vi "Can软件版本号.vi"() -> (3 "软件版本号":string)   [LabVIEW 2020]
uses:
  Libraries/ZLG_CAN/ZLG_CAN.lvlib
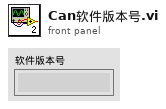
[diagram p1: front panel]
types:
  T1 = typedef "ZLG_CAN.lvlib/CAN_Frame.ctl" = cluster{"[0]":u8, "[1]":u8, "[2]":u8, "[3]":u8, "[4]":u8, "[5]":u8, "[6]":u8, "[7]":u8}
  T2 = typedef "ZLG_CAN.lvlib/Sent_Recive (Reply Payload)--cluster.ctl" = cluster{"Receive":T3[], "Sent_Recive_error":errorcluster}
  T3 = typedef "ZLG_CAN.lvlib/CAN_OBJ_R.ctl" = cluster{"ID":u32, "TimeStamp":u32, "TimeFlag":u8, "SendType":u8, "RemoteFlag":u8, "ExternFlag":u8, "DataLen":u8, "数值":u8, "数值":u8, "数值":u8, "数值":u8, "数值":u8, "数值":u8, "数值":u8, "数值":u8, "数值":u8, "数值":u8, "数值":u8}
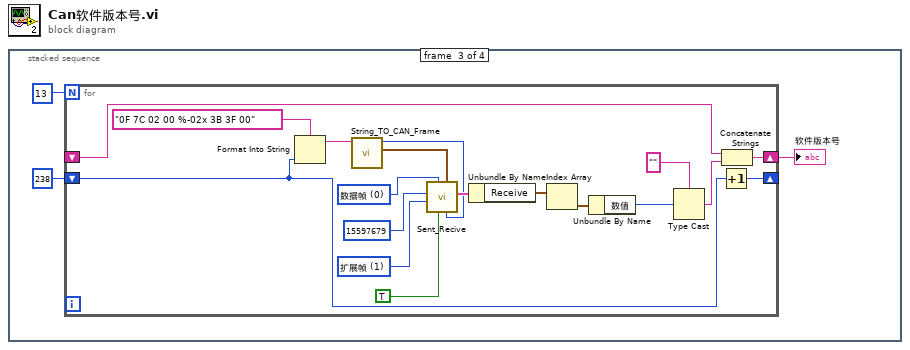
[diagram p0: block diagram]
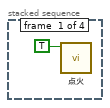
[diagram p2: hidden frame]
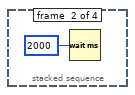
[diagram p3: hidden frame]
diagram:
  n1 = stacked-sequence {
    frame #0 {
      n2 = call "点火.vi"("点火"=TRUE) -> ()  [unwired: 10 in, 1 out]
    }
    frame #1 {
      n3 = Wait (ms)(milliseconds to wait=u32 2000 ("等待时间（毫秒）")) -> ()  [unwired: 1 out]
    }
    frame #2 {
      n4 = for {
        N: 13 -> [_]
        shift-right: [w16] -> _
        shift-left: u8 238 -> [w17]
        shift-right: [w7] -> w3
        shift-left: _ -> [w6]
        w22 = u8 1 items=["标准帧", "扩展帧"] ("帧类型")
        w23 = u8 0 items=["数据帧", "远程帧"] ("帧格式")
        n5 = Format Into String(format string="0F 7C 02 00 %-02x 3B 3F 00" ("格式字符串"), w17) -> (resulting string=w19:string)  [unwired: 2 in, 1 out]
        n6 = call "String_TO_CAN_Frame.vi"("CAN_Frame"=w19) -> ("CAN_FRAME"=w15:T1, "DATA_LEN"=w14:i32)  [unwired: 9 in]
        n7 = call "Sent_Recive.vi"("帧长度"=w14, "CAN_FRAME"=w15, "wait for reply (T)"=TRUE, "帧格式"=w23, "帧类型"=w22, "ID"=u32 15597679) -> ("Reply Payload"=w20:T2)  [unwired: 3 in, 2 out]
        n8 = Unbundle By Name(w20) -> ("Receive"=w13:T3[])
        n9 = Index Array(array=w13) -> (element=w12:T3)  [unwired: 1 in]
        n10 = Unbundle By Name(w12) -> ("数值"=w10:u8)
        n11 = Type Cast(type="", x=w10) -> (*(type *) &x=w9:string)
        n12 = Increment(x=w17) -> (x+1=w16:u8)
        n13 = Concatenate Strings(w6, w9) -> (w7:string)
      }
      "软件版本号" <- w3
    }
    frame #3 {
    }
  }
